vi "Andor_iXon_GetData_Point-Picture.vi"(8 "Input Cluster":T6, 11 "Measure":bool) -> (0 "Output Cluster":T6)   [LabVIEW 2009]
uses:
  atmcd32d.llb/AcquisitionMode_mode typedef.ctl
  atmcd32d.llb/ReadMode_mode typedef.ctl
  atmcd32d.llb/TriggerMode_mode typedef.ctl
  atmcd32d.llb/Shutter_type typedef.ctl
  atmcd32d.llb/Shutter_mode typedef.ctl
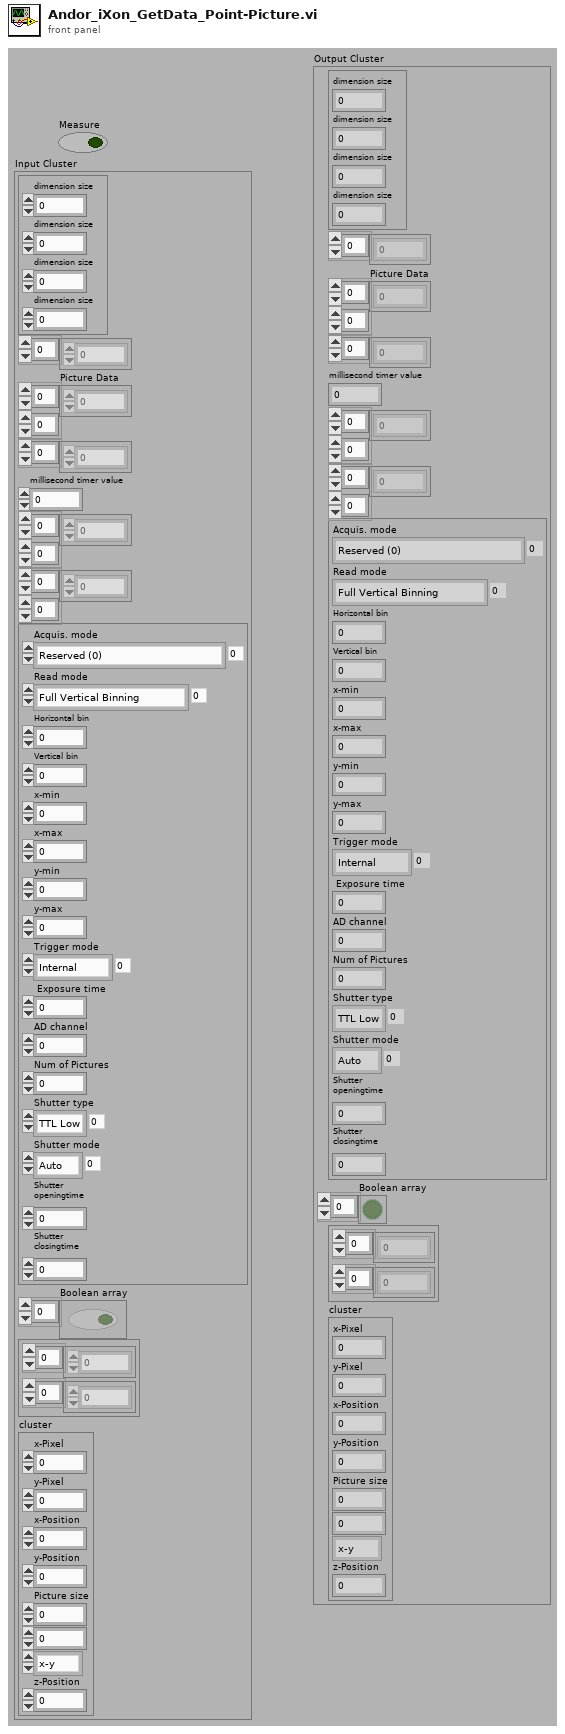
[diagram p1: front panel]
types:
  T1 = typedef "AcquisitionMode_mode typedef.ctl" = enum16{"Reserved (0)", "Single Scan", "Accumulate", "Kinetics", "Fast Kinetics", "Run Till Abort", "Reserved (6)", "Reserved (7)", "Reserved (8)", "Time Delayed Integration"}
  T2 = typedef "ReadMode_mode typedef.ctl" = enum16{"Full Vertical Binning", "Multi-Track", "Random-Track", "Single-Track", "Image"}
  T3 = typedef "TriggerMode_mode typedef.ctl" = enum16{"Internal", "External", "N/A (2)", "N/A (3)", "N/A (4)", "N/A (5)", "External Start"}
  T4 = typedef "Shutter_type typedef.ctl" = enum16{"TTL Low", "TTL High"}
  T5 = typedef "Shutter_mode typedef.ctl" = enum16{"Auto", "Open", "Close"}
  T6 = cluster{cluster{"dimension size":i32, "dimension size":i32, "dimension size":i32, "dimension size":i32}, i32[], "Picture Data":dbl[][], u32[], "millisecond timer value":u32, dbl[][], i32[][], cluster{"Acquis. mode":T1, "Read mode":T2, "Horizontal bin":i32, "Vertical bin":i32, "x-min":i32, "x-max":i32, "y-min":i32, "y-max":i32, "Trigger mode":T3, " Exposure time":sgl, "AD channel":i32, "Num of Pictures":i32, "Shutter type":T4, "Shutter mode":T5, "Shutter\nopeningtime":i32, "Shutter\nclosingtime":i32}, "Boolean array":bool[], cluster{dbl[], dbl[]}, "cluster":cluster{"x-Pixel":u16, "y-Pixel":u16, "x-Position":dbl, "y-Position":dbl, "Picture size":dbl, dbl, enum32{"x-y", "x-z", "y-z"}, "z-Position":dbl}}
  T7 = cluster{"Acquis. mode":T1, "Read mode":T2, "Horizontal bin":i32, "Vertical bin":i32, "x-min":i32, "x-max":i32, "y-min":i32, "y-max":i32, "Trigger mode":T3, " Exposure time":sgl, "AD channel":i32, "Num of Pictures":i32, "Shutter type":T4, "Shutter mode":T5, "Shutter\nopeningtime":i32, "Shutter\nclosingtime":i32}
  T8 = typedef "Error Code Enum typedef.ctl" = enum32{"N/A (0)", "DRV_ERROR_CODES", "DRV_SUCCESS", "DRV_VXDNOTINSTALLED", "DRV_ERROR_SCAN", "DRV_ERROR_CHECK_SUM", "DRV_ERROR_FILELOAD", "DRV_UNKNOWN_FUNC", "DRV_ERROR_VXD_INIT", "DRV_ERROR_ADDRESS", "DRV_ERROR_PAGELOCK", "DRV_ERROR_PAGEUNLOCK", "DRV_ERROR_BOARDTEST", "DRV_ERROR_ACK", "DRV_ERROR_UP_FIFO", "DRV_ERROR_PATTERN", "N/A (16)", "DRV_ACQUISITION_ERRORS", "DRV_ACQ_BUFFER", "DRV_ACQ_DOWNFIFO_FULL", "DRV_PROC_UNKONWN_INSTRUCTION", "DRV_ILLEGAL_OP_CODE", "DRV_KINETIC_TIME_NOT_MET", "DRV_ACCUM_TIME_NOT_MET", "DRV_NO_NEW_DATA", "N/A (25)", "DRV_SPOOLERROR", "N/A (27)", "N/A (28)", "N/A (29)", "N/A (30)", "N/A (31)", "N/A (32)", "DRV_TEMPERATURE_CODES", "DRV_TEMPERATURE_OFF", "DRV_TEMPERATURE_NOT_STABILIZED", "DRV_TEMPERATURE_STABILIZED", "DRV_TEMPERATURE_NOT_REACHED", "DRV_TEMPERATURE_OUT_RANGE", "DRV_TEMPERATURE_NOT_SUPPORTED", "DRV_TEMPERATURE_DRIFT", "N/A (41)", "N/A (42)", "N/A (43)", "N/A (44)", "N/A (45)", "N/A (46)", "N/A (47)", "N/A (48)", "DRV_GENERAL_ERRORS", "DRV_INVALID_AUX", "DRV_COF_NOTLOADED", "DRV_FPGAPROG", "DRV_FLEXERROR", "DRV_GPIBERROR", "N/A (55)", "N/A (56)", "N/A (57)", "N/A (58)", "N/A (59)", "N/A (60)", "N/A (61)", "N/A (62)", "N/A (63)", "DRV_DATATYPE", "DRV_DRIVER_ERRORS", "DRV_P1INVALID", "DRV_P2INVALID", "DRV_P3INVALID", "DRV_P4INVALID", "DRV_INIERROR", "DRV_COFERROR", "DRV_ACQUIRING", "DRV_IDLE", "DRV_TEMPCYCLE", "DRV_NOT_INITIALIZED", "DRV_P5INVALID", "DRV_P6INVALID", "DRV_INVALID_MODE", "DRV_INVALID_FILTER", "DRV_I2CERRORS", "DRV_I2CDEVNOTFOUND", "DRV_I2CTIMEOUT", "DRV_P7INVALID", "N/A (84)", "N/A (85)", "N/A (86)", "N/A (87)", "N/A (88)", "N/A (89)", "DRV_IOCERROR", "DRV_VRMVERSIONERROR"}
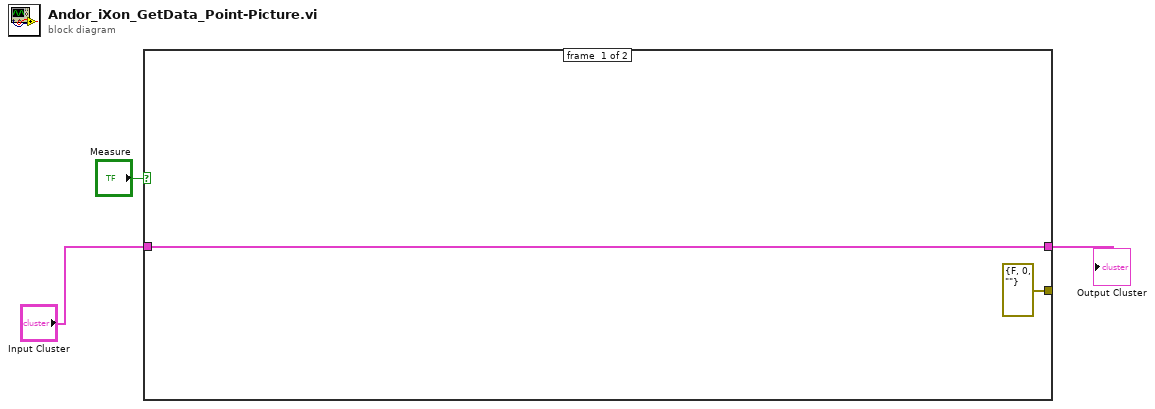
[diagram p0: block diagram]
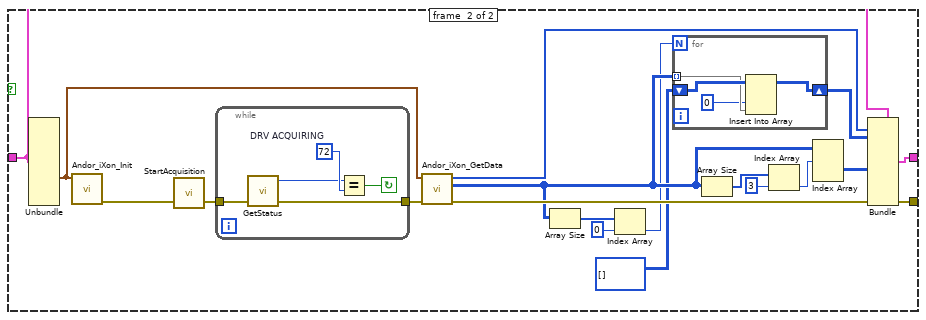
[diagram p2: hidden frame]
diagram:
  n1 = case shown="True" "Measure" {
    tunnel: "Input Cluster" -> [w5 w17]
    tunnel: [w5 w22] -> w2
    tunnel: [errorcluster {"status"=FALSE, "code"=0, "source"=""} ("error out") w19] -> _
    frame #0 {
    }
    frame #1 {
      n2 = Unbundle(w17) -> (w15:T7)  [unwired: 10 out]
      n3 = call "Andor_iXon_Init.vi"("input cluster"=w15) -> ("error out"=w16:errorcluster)  [unwired: 1 in, 9 out]
      n4 = call "StartAcquisition.vi"("error in (no error)"=w16) -> ("error out"=w18:errorcluster)  [unwired: 2 out]
      n5 = while {
        tunnel: [w29] -> w23
        tunnel: w18 -> [w28]
        stop <- w31 continue-if-true
        w32 = u16 72  # DRV ACQUIRING
        n6 = call "GetStatus.vi"("error in (no error)"=w28) -> ("error out"=w29:errorcluster, "status"=w30:T8)  [unwired: 3 out]
        n7 = Equal?(x=w30, y=w32) -> (x = y?=w31:bool)
      }
      n8 = call "Andor_iXon_GetData.vi"("error in"=w23, "input cluster"=w15) -> ("error out"=w19:errorcluster, "Array 3"=w11:i32[][][], "array"=w14:i32[])  [unwired: 2 in, 5 out]
      n9 = Array Size(array=w11) -> (size(s)=w13:i32[])
      n10 = Index Array(array=w13, index=0) -> (element=w9:i32)
      n11 = for {
        N: w9 -> [_]
        tunnel: w11 -> [w25] mode=indexing
        shift-right: [w26] -> w8
        shift-left: i32[][] [] ("subarray") -> [w27]
        n12 = Insert Into Array(array=w27, index (col)=0 ("disabled index (col)"), new element=w25) -> (w26:i32[][])  [unwired: 1 in]
      }
      n13 = Array Size(array=w11) -> (size(s)=w21:i32[])
      n14 = Index Array(array=w21, index=3) -> (element=w10:i32)
      n15 = Index Array(array=w11, index (dim 0)=w10) -> (element=w7:i32[][])  [unwired: 2 in]
      n16 = Bundle(cluster=w17, w14, "Picture Data"=w8, w7) -> (w22:T6)  [unwired: 8 out]
    }
  }
  "Output Cluster" <- w2
